vi "GetDFromB.vi"(1 "Control":bool, 2 "ArrayIn":waveform(i16)[](array[waveform]), 3 "Bool Refnum":refnum<vi>) -> (0 "ArrayOut":waveform(i16)[](array[waveform]))   [LabVIEW 2010]
uses:
  70user.lib/TheSigTab.vi
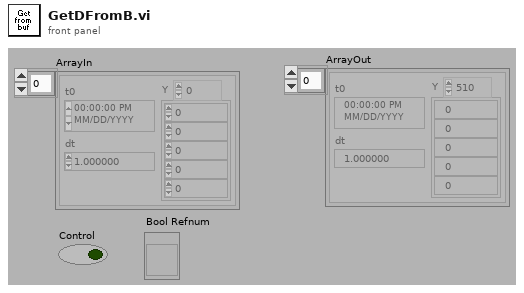
[diagram p1: front panel]
types:
  T1 = cluster{"Status":bool, "ViErrorNumber":u32, "ViName":string, "ViErrorString":string, "CinName":string, "CinErrorString":string}
  T2 = cluster{"DllVersion":u32, "InterfaceType":u32, "InterfaceInstance":u32, "ModuleHandle":u32, "ReadBuffersParsArray":cluster{"Buffer":i16[], "ReadOv":u32, "ReadEvent":u32}[], "WriteBuffersParsArray":cluster{"Buffer":i16[], "WriteOv":u32, "WriteEvent":u32}[]}
  T3 = cluster{u32, "BufSize":u32, "RequestStatus":bool}
  T4 = cluster{"ReadBufferIndex":u32, "NumberOfWordsToRead":u32, "RequestStatus":bool}
  T5 = cluster{"Buffer":i16[], "ReadOv":u32, "ReadEvent":u32}[]
  T6 = cluster{"s_Type":u16, "FIFO":u16, "IrqStep":u16, "Pages":u16, "AutoInit":u16, "dRate":dbl, "dKadr":dbl, "dScale":dbl, "Rate":u16, "Kadr":u16, "Scale":u16, "FPDelay":u16, "SynchroType":u16, "SynchroSensitivity":u16, "SynchroMode":u16, "AdChannel":u16, "AdPorog":u16, "NCh":u16, "Chn":i32[], "IrqEna":u16, "AdcEna":u16}
  T7 = cluster{"Buffer":i16[], "ReadOv":u32, "ReadEvent":u32}
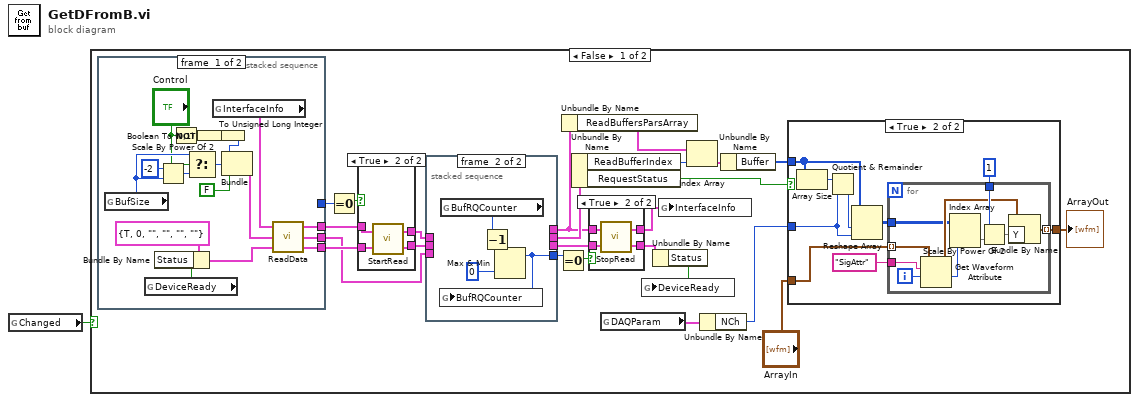
[diagram p0: block diagram]
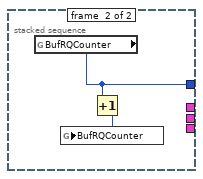
[diagram p2: hidden frame]
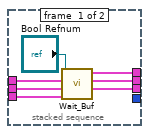
[diagram p3: hidden frame]
diagram:
  n1 = global read "TheSigTab.vi" "Changed"() -> (w1:bool)
  n2 = case shown="False" w1 {
    frame False {
      n3 = stacked-sequence {
        tunnel: [w31 _] -> w14
        tunnel: [w30 _] -> w15
        tunnel: [w29 _] -> w16
        tunnel: [_ w43] -> w25
        frame #0 {
          n4 = global read "TheSigTab.vi" "BufSize"() -> (w36:u32)
          n5 = global read "TheSigTab.vi" "DeviceReady"() -> (w32:bool)
          n6 = Bundle By Name(cluster=T1 {"Status"=TRUE, "ViErrorNumber"=0, "ViName"="", "ViErrorString"="", "CinName"="", "CinErrorString"=""} ("ViStatusIn"), "Status"=w32) -> (w27:T1)
          n7 = Scale By Power Of 2(n=-2, x=w36) -> (x*2^n=w37:u32)
          n8 = Not(x="Control") -> (.not. x?=w38:bool)
          n9 = Select(t=w36, s="Control", f=w37) -> (s? t:f=w35:u32)
          n10 = Boolean To (0,1)(Boolean=w38) -> (0, 1=w42:i16)
          n11 = global read "TheSigTab.vi" "InterfaceInfo"() -> (w28:T2)
          n12 = To Unsigned Long Integer(number=w42) -> (unsigned 32bit integer=w39:u32)
          n13 = Bundle(w39, "BufSize"=w35, "RequestStatus"=FALSE) -> (w26:T3)  [unwired: 1 in]
          n14 = call "ReadData.vi"("ViStatusIn"=w27, "ReadParsIn"=w26, "InterfaceInfoIn"=w28) -> ("ViStatusOut"=w29:T1, "ReadParsOut"=w31:T4, "InterfaceInfoOut"=w30:T2)
        }
        frame #1 {
          n15 = global read "TheSigTab.vi" "BufRQCounter"() -> (w43:i32)
          n16 = Increment(x=w43) -> (x+1=w44:i32)
          n17 = global write "TheSigTab.vi" "BufRQCounter"(w44) -> ()
        }
      }
      n18 = Equal To 0?(x=w25) -> (x = 0?=w17:bool)
      n19 = case shown="True" w17 {
        tunnel: [w56 w61] -> w11
        tunnel: [w57 w60] -> w12
        tunnel: w15 -> [w56 w59]
        tunnel: w16 -> [w57 w58]
        frame False {
        }
        frame True {
          n20 = call "StartRead.vi"("ViStatusIn"=w58, "InterfaceInfoIn"=w59) -> ("ViStatusOut"=w60:T1, "InterfaceInfoOut"=w61:T2)
        }
      }
      n21 = stacked-sequence {
        tunnel: [w51 _] -> w5
        tunnel: [w50 _] -> w8
        tunnel: [w49 _] -> w10
        tunnel: w11 -> [w48 _]
        tunnel: w12 -> [w47 _]
        tunnel: w14 -> [w46 _]
        tunnel: [_ w52] -> w24
        frame #0 {
          n22 = call "Wait_Buf.vi"("ReadParsIn"=w46, "ViStatusIn"=w47, "InterfaceInfoIn"=w48, "reference"="Bool Refnum") -> ("ViStatusOut"=w50:T1, "ReadPars"=w49:T4, "InterfaceInfoOut"=w51:T2)  [unwired: 2 in]
        }
        frame #1 {
          n23 = global read "TheSigTab.vi" "BufRQCounter"() -> (w55:i32)
          n24 = Decrement(x=w55) -> (x-1=w53:i32)
          n25 = Max & Min(x=w53, y=0) -> (max(x,y)=w52:i32)  [unwired: 1 out]
          n26 = global write "TheSigTab.vi" "BufRQCounter"(w52) -> ()
        }
      }
      n27 = Equal To 0?(x=w24) -> (x = 0?=w18:bool)
      n28 = Unbundle By Name(w5) -> ("ReadBuffersParsArray"=w7:T5)
      n29 = Unbundle By Name(w10) -> ("ReadBufferIndex"=w9:u32, "RequestStatus"=w13:bool)
      n30 = case shown="True" w18 {
        tunnel: w5 -> [w63 w67]
        tunnel: [w63 w66] -> w23
        tunnel: w8 -> [w62 w65]
        tunnel: [w62 w64] -> w22
        frame False {
        }
        frame True {
          n31 = call "StopRead.vi"("ViStatusIn"=w65, "InterfaceInfoIn"=w67) -> ("ViStatusOut"=w64:T1, "InterfaceInfoOut"=w66:T2)
        }
      }
      n32 = global read "TheSigTab.vi" "DAQParam"() -> (w2:T6)
      n33 = Unbundle By Name(w22) -> ("Status"=w3:bool)
      n34 = global write "TheSigTab.vi" "DeviceReady"(w3) -> ()
      n35 = global write "TheSigTab.vi" "InterfaceInfo"(w23) -> ()
      n36 = Index Array(array=w7, index=w9) -> (element=w6:T7)
      n37 = Unbundle By Name(w2) -> ("NCh"=w19:u16)
      n38 = Unbundle By Name(w6) -> ("Buffer"=w4:i16[])
      n39 = case shown="True" w13 {
        tunnel: w4 -> [_ w76]
        tunnel: [w68 w74] -> w21
        tunnel: "ArrayIn" -> [w68 w73]
        tunnel: w19 -> [_ w69]
        frame False {
        }
        frame True {
          n40 = Array Size(array=w76) -> (size(s)=w75:i32)
          n41 = Quotient & Remainder(x=w75, y=w69) -> (floor(x/y)=w77:i32)  [unwired: 1 out]
          n42 = Reshape Array(w76, w77, w69) -> (w71:i16[][])
          n43 = for {
            tunnel: w73 -> [w84] mode=indexing
            tunnel: [w87] -> w74 mode=indexing
            tunnel: w71 -> [w82]
            tunnel: 1 -> [w85]
            tunnel: "SigAttr" -> [w80]
            i -> [w79]
            n44 = Get Waveform Attribute(5:w79, 6:w80, 7:w84) -> (1:w78:i32, 3:w83:waveform(i16))  [unwired: 1 in, 2 out]
            n45 = Index Array(array=w82, index (col)=w78) -> (element=w81:i16[])  [unwired: 1 in]
            n46 = Scale By Power Of 2(n=w85, x=w81) -> (x*2^n=w86:i16[])
            n47 = Bundle By Name(cluster=w83, "Y"=w86) -> (w87:waveform(i16))
          }
        }
      }
      "ArrayOut" <- w21
    }
    frame True {
    }
  }
